vi "DCA Handle Test Complete.vi"(6 "Quick Mode (F)":bool, 8 "error in (no error)":errorcluster, 9 "Test Parameters":T1={"Stimulus"={"Use Instrument"=FALSE, "Normalize"=FALSE, "Blank Screen"=FALSE, "Measurement Type"=enum."Voltage DC", "Range"=enum."Auto", "Resolution"=enum."Auto"}, "Measurement"={"Topology"=enum."PI-Network", "Lock Topology"=FALSE, "ATTN Calc"=enum."Power", "Zo"=50.0}, "Limits"=[], "Normalization"={"Normalized?"=FALSE, "Rab Value"=0.0, "Rac Value"=0.0, "Rbc Value"=0.0}}, 11 "Queue":refnum<queue>) -> (0 "error out":errorcluster)   [LabVIEW 2011]
uses:
  TypeDefs/DCA Queue Cluster.ctl
  TypeDefs/DCA Test Parameters.ctl
  TypeDefs/DCA Stimulus Parameters.ctl
  TypeDefs/DCA Measurement Cluster.ctl
  TypeDefs/DCA Topology.ctl
  TypeDefs/DCA Attenuation Calculation.ctl
  TypeDefs/DCA Limit.ctl
  TypeDefs/DCA Limit Quantity.ctl
  TypeDefs/DCA Limit Comparison.ctl
  TypeDefs/DCA Limit Operation.ctl
  Test Referential Limit.ctl
  TypeDefs/DCA Calibration State.ctl
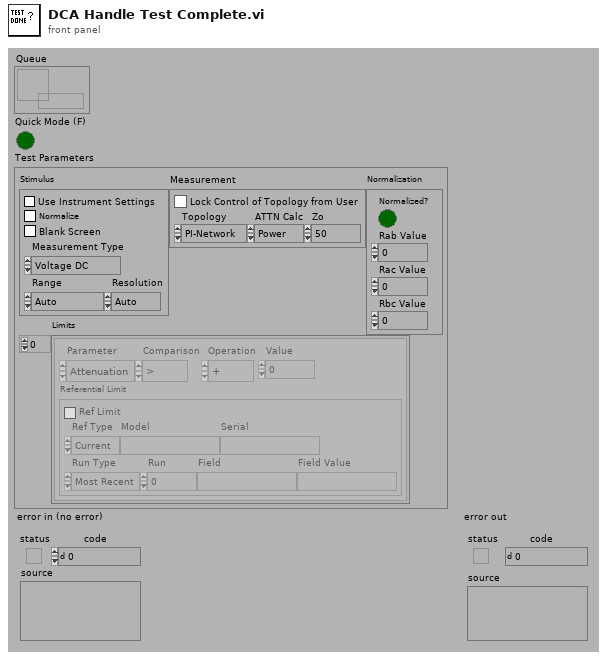
[diagram p1: front panel]
types:
  T1 = typedef "DCA Test Parameters.ctl" = cluster{"Stimulus":T2, "Measurement":T3, "Limits":T6[], "Normalization":T11}
  T2 = typedef "DCA Stimulus Parameters.ctl" = cluster{"Use Instrument":bool, "Normalize":bool, "Blank Screen":bool, "Measurement Type":enum16{"Voltage DC", "Voltage DC Ratio", "Voltage AC", "Current DC", "Current AC", "Resistance", "Fresistance", "Frequency", "Period", "Continuity", "Diode"}, "Range":enum16{"Auto", "Minimum", "Maximum", "100", "1,000", "10,000", "100,000", "1,000,000", "10,000,000", "100,000,000"}, "Resolution":enum16{"Auto", "4 1/2", "5 1/2", "6 1/2"}}
  T3 = typedef "DCA Measurement Cluster.ctl" = cluster{"Topology":T4, "Lock Topology":bool, "ATTN Calc":T5, "Zo":dbl}
  T4 = typedef "DCA Topology.ctl" = enum32{"PI-Network", "T-Network"}
  T5 = typedef "DCA Attenuation Calculation.ctl" = enum32{"Power", "Voltage"}
  T6 = typedef "DCA Limit.ctl" = cluster{"Parameter":T7, "Comparison":T8, "Operation":T9, "Value":dbl, "Referential Limit":T10}
  T7 = typedef "DCA Limit Quantity.ctl" = enum16{"Attenuation", "Zin", "Zout", "R1", "R2", "R3", "Rab", "Rac", "Rbc"}
  T8 = typedef "DCA Limit Comparison.ctl" = enum16{">", ">=", "<", "<="}
  T9 = typedef "DCA Limit Operation.ctl" = enum16{"+", "-"}
  T10 = typedef "Test Referential Limit.ctl" = cluster{"Ref Limit":bool, "Ref Type":enum16{"Current", "Specify"}, "Model":string, "Serial":string, "Run Type":enum16{"Most Recent", "Run #", "Match Field"}, "Run":i32, "Field":string, "Field Value":string}
  T11 = typedef "DCA Calibration State.ctl" = cluster{"Normalized?":bool, "Rab Value":dbl, "Rac Value":dbl, "Rbc Value":dbl}
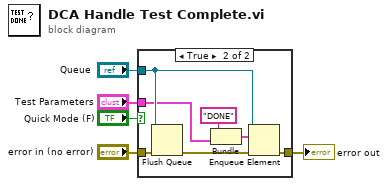
[diagram p0: block diagram]
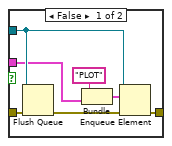
[diagram p2: hidden frame]
diagram:
  n1 = case shown="True" "Quick Mode (F)" {
    tunnel: [w12 w19] -> w5
    tunnel: "Queue" -> [w8 w15]
    tunnel: "error in (no error)" -> [w9 w16]
    tunnel: "Test Parameters" -> [w6 w13]
    frame False {
      n2 = Flush Queue(queue=w8, error in (no error)=w9) -> (error out=w7:errorcluster)  [unwired: 2 out]
      n3 = Bundle("PLOT", "Test Parameters"=w6) -> (w10:cluster{string, "Test Parameters":T1})  [unwired: 1 out]
      n4 = Enqueue Element(queue=w8, element=w10, error in (no error)=w7) -> (error out=w12:errorcluster)  [unwired: 3 out]
    }
    frame True {
      n5 = Flush Queue(queue=w15, error in (no error)=w16) -> (error out=w14:errorcluster)  [unwired: 2 out]
      n6 = Bundle("DONE", "Test Parameters"=w13) -> (w17:cluster{string, "Test Parameters":T1})  [unwired: 1 out]
      n7 = Enqueue Element(queue=w15, element=w17, error in (no error)=w14) -> (error out=w19:errorcluster)  [unwired: 3 out]
    }
  }
  "error out" <- w5
